vi "FGV Status Analysatoren.vi"(6 "Aktionen":T3, 7 "Controls[]":refnum<vi>[](array[refnum]), 9 "Fehler":bool, 10 "Aktiv":T2) -> (2 "Status Analysatoren":T1)   [LabVIEW 2020, in "Status Analysatoren.lvlib"]
uses:
  Status Analysatoren.lvlib
  Aktion Status Analysatoren.ctl
  Status Analysatoren_Anzeige.ctl
  Status.ctl
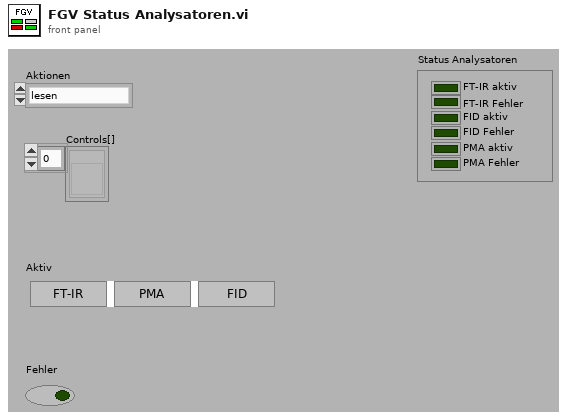
[diagram p1: front panel]
types:
  T1 = typedef "Status Analysatoren.lvlib/Status.ctl" = cluster{"FT-IR aktiv":bool, "FT-IR Fehler":bool, "FID aktiv":bool, "FID Fehler":bool, "PMA aktiv":bool, "PMA Fehler":bool}
  T2 = typedef "Status Analysatoren.lvlib/Status Analysatoren_Anzeige.ctl" = cluster{"FT-IR":bool, "FID":bool, "PMA":bool}
  T3 = typedef "Status Analysatoren.lvlib/Aktion Status Analysatoren.ctl" = enum16{"lesen", "initialisieren", "Analysatoren aktiv", "FTIR Fehler", "FID Fehler", "PMA Fehler", "Felder einfärben"}
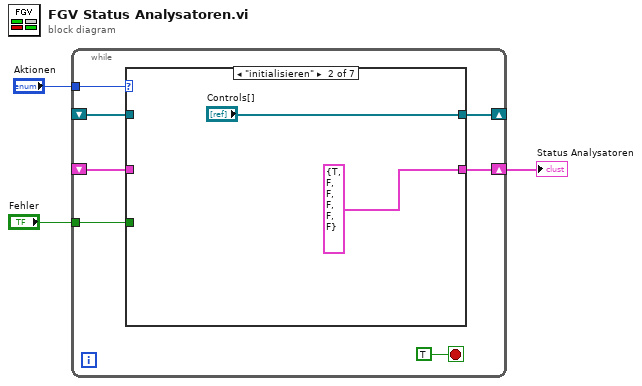
[diagram p0: block diagram]
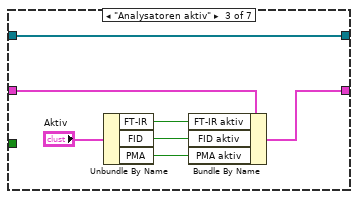
[diagram p3: hidden frame]
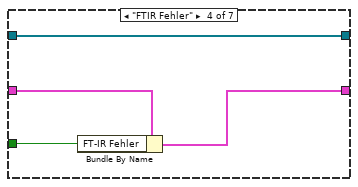
[diagram p4: hidden frame]
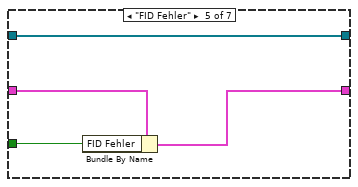
[diagram p5: hidden frame]
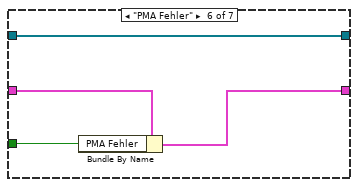
[diagram p6: hidden frame]
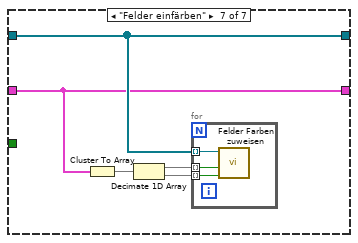
[diagram p7: hidden frame]
diagram:
  n1 = while {
    tunnel: "Aktionen" -> [w10]
    shift-right: [w9] -> _
    shift-left: _ -> [w8]
    tunnel: "Fehler" -> [w7]
    shift-right: [w5] -> w1
    shift-left: _ -> [w4]
    stop <- TRUE stop-if-true
    n2 = case shown="\"initialisieren\"" w10 {
      tunnel: [w12 "Controls[]" w21 w25 w29 w33 w38] -> w9
      tunnel: w8 -> [w12 _ w21 w25 w29 w33 w38]
      tunnel: w7 -> [_ _ _ w23 w27 w31 _]
      tunnel: [w11 T1 {"FT-IR aktiv"=TRUE, "FT-IR Fehler"=FALSE, "FID aktiv"=FALSE, "FID Fehler"=FALSE, "PMA aktiv"=FALSE, "PMA Fehler"=FALSE} ("Status Analysatoren") w17 w22 w26 w30 w34] -> w5
      tunnel: w4 -> [w11 _ w20 w24 w28 w32 w34]
      frame "lesen", Default {
      }
      frame "initialisieren" {
      }
      frame "Analysatoren aktiv" {
        n3 = Unbundle By Name("Aktiv") -> ("FT-IR"=w19:bool, "FID"=w18:bool, "PMA"=w15:bool)
        n4 = Bundle By Name(cluster=w20, "FT-IR aktiv"=w19, "FID aktiv"=w18, "PMA aktiv"=w15) -> (w17:T1)
      }
      frame "FTIR Fehler" {
        n5 = Bundle By Name(cluster=w24, "FT-IR Fehler"=w23) -> (w22:T1)
      }
      frame "FID Fehler" {
        n6 = Bundle By Name(cluster=w28, "FID Fehler"=w27) -> (w26:T1)
      }
      frame "PMA Fehler" {
        n7 = Bundle By Name(cluster=w32, "PMA Fehler"=w31) -> (w30:T1)
      }
      frame "Felder einfärben" {
        n8 = Cluster To Array(cluster=w34) -> (array=w37:bool[])
        n9 = Decimate 1D Array(w37) -> (w36:bool[], w35:bool[])
        n10 = for {
          tunnel: w38 -> [w41] mode=indexing
          tunnel: w36 -> [w40] mode=indexing
          tunnel: w35 -> [w39] mode=indexing
          n11 = call "Felder Farben zuweisen.vi"("Fehler"=w39, "Aktiv"=w40, "Element"=w41) -> ()  [unwired: 9 in]
        }
      }
    }
  }
  "Status Analysatoren" <- w1
